vi "Measurement Logic.vi"() -> ()   [LabVIEW 2021, in "Stepped Frequency Sweep_Audio DAC.lvlib"]
uses:
  Stepped Frequency Sweep_Audio DAC.lvlib
  <vilib>/PDM Acquisition Toolkit/host/Classes/Channels/I2S Ouput/Controls/GenerationChannelProperties.ctl
  <vilib>/PDM Acquisition Toolkit/host/Classes/Channels/I2S Ouput/I2S Output Channel.lvclass
  <vilib>/PDM Acquisition Toolkit/host/Classes/Tasks/I2S Output/Control/SignalProperties.ctl
  <vilib>/PDM Acquisition Toolkit/host/Classes/Tasks/I2S Output/I2S Output Task.lvclass
  shared/controls/Digital Initialize Settings.ctl
  shared/controls/Analog Initialize Settings.ctl
  shared/controls/Single Tone Measurement Settings.ctl
  shared/controls/Single Tone Units.ctl
  Measurement Results.ctl
  <vilib>/Analysis/NI_AALBase.lvlib
  <vilib>/Analysis/1siggen.llb/Ramp Pattern by Samples.vi
  <vilib>/MeasurementLink/MeasurementLink Measurement Server/Measure Call Context/Measure Call Context.lvclass
  shared/controls/Single Tone Filter Settings.ctl
  Measurement Configuration.ctl
panel:
  out "measure call context out":refnum<class "Measure Call Context.lvclass">
  in  "measure call context in":refnum<class "Measure Call Context.lvclass">
  out "measurement results":T1 {"Gain" format="%_6g"; "THD" format="%_6g"; "THD+N" format="%_6g"; "SNR" format="%_6g"; "SFDR (dBc)" format="%_6g"; "Dynamic range (dB)" format="%_6g"; "Phase (deg)" format="%_6g"; "Amplitude (dB)" format="%_6g"; "Amplitude (V)" format="%_6g"; "Frequency (Hz)" format="%_6g"; "df" format="%_6g"; "f0" format="%_6g"; "dt" format="%_6g"; "Frequency domain" format="%_6g"; "Time domain" format="%_6g"}
  in  "measurement configuration":T2={"Protocol file"="", "Digital audio channel"="", "Master clock channel"="", "Sweep Start (Hz)"=1000.0, "Sweep Stop (Hz)"=20000.0, "Sweep Steps"=11, "Sweep Profile"="Logarithmic", "Output level"=-1.0, "Output level units"="", "Output range (Vpk-pk)"=15.0, "Acquisition channel"="", "Sample rate (Hz)"=51200.0, "Min measurement cycles"=0, "Min measurement time (s)"=0.1, "Min settling cycles"=0, "Min settling time (s)"=0.1, "Band start (Hz)"=20.0, "Band stop (Hz)"=20000.0, "SNR units"="", "THD+N units"="", "THD units"="", "Gain units"="", "Highpass filter"="", "Lowpass filter"="", "Weighting filter"=""} {"Sweep Stop (Hz)" format="%#_6pHz"; "Band stop (Hz)" format="%#_6pHz"; "Band start (Hz)" format="%#_6pHz"; "Min settling time (s)" format="%#_6ps"; "Min measurement time (s)" format="%#_6ps"; "Sample rate (Hz)" format="%#_6pHz"; "Output range (Vpk-pk)" format="%.3p Vpk-pk"; "Output level" format="%#_6p"; "Sweep Start (Hz)" format="%#_6pHz"}
  out "error out":errorcluster
  in  "error in":errorcluster
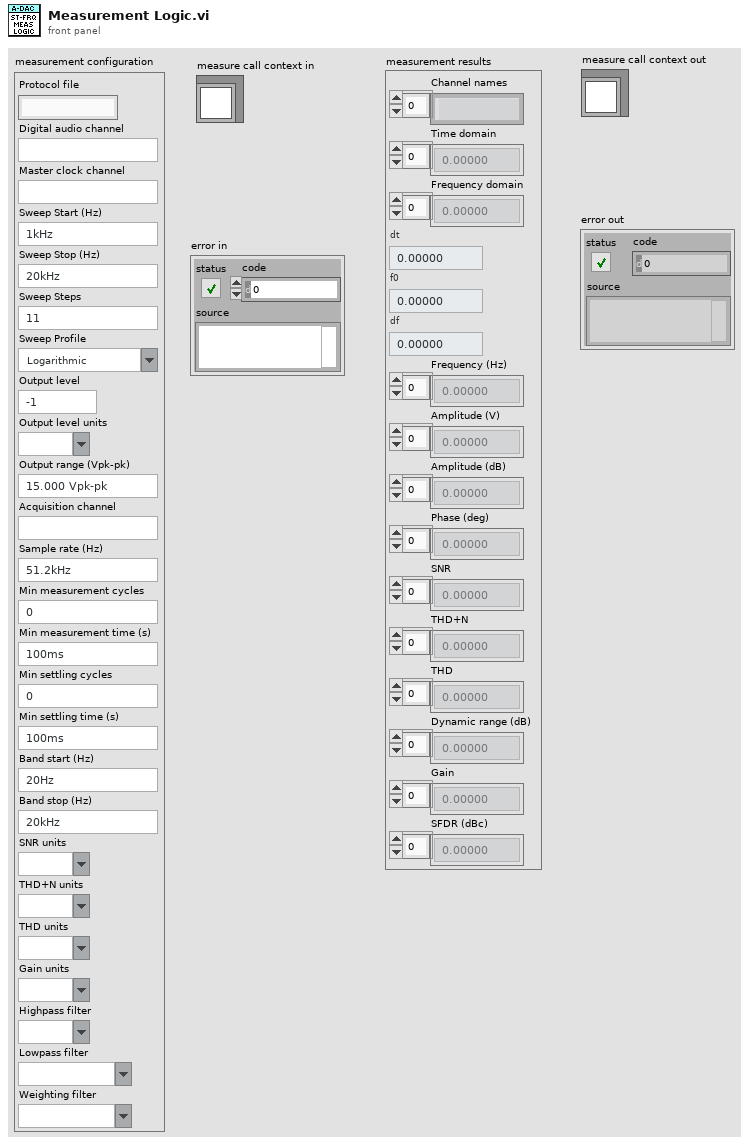
[diagram p1: front panel]
types:
  T1 = typedef "Stepped Frequency Sweep_Audio DAC.lvlib/Measurement Results.ctl" = cluster{"Channel names":string[], "Time domain":dbl[], "Frequency domain":dbl[], "dt":dbl, "f0":dbl, "df":dbl, "Frequency (Hz)":dbl[], "Amplitude (V)":dbl[], "Amplitude (dB)":dbl[], "Phase (deg)":dbl[], "SNR":dbl[], "THD+N":dbl[], "THD":dbl[], "Dynamic range (dB)":dbl[], "Gain":dbl[], "SFDR (dBc)":dbl[]}
  T2 = typedef "Stepped Frequency Sweep_Audio DAC.lvlib/Measurement Configuration.ctl" = cluster{"Protocol file":string, "Digital audio channel":string, "Master clock channel":string, "Sweep Start (Hz)":dbl, "Sweep Stop (Hz)":dbl, "Sweep Steps":u32, "Sweep Profile":string, "Output level":dbl, "Output level units":string, "Output range (Vpk-pk)":dbl, "Acquisition channel":string, "Sample rate (Hz)":dbl, "Min measurement cycles":u32, "Min measurement time (s)":dbl, "Min settling cycles":u32, "Min settling time (s)":dbl, "Band start (Hz)":dbl, "Band stop (Hz)":dbl, "SNR units":string, "THD+N units":string, "THD units":string, "Gain units":string, "Highpass filter":string, "Lowpass filter":string, "Weighting filter":string}
  T3 = typedef "Single Tone Filter Settings.ctl" = cluster{"Highpass filter":string, "Lowpass filter":string, "Weighting filter":string}
  T4 = typedef "Single Tone Units.ctl" = cluster{"SNR units":string, "THD+N units":string, "THD units":string, "Gain units":string}
  T5 = typedef "Single Tone Measurement Settings.ctl" = cluster{"Band start":dbl, "Band stop":dbl, "Amplitude":dbl, "Frequency":dbl, "Full scale range":dbl}
  T6 = typedef "Analog Initialize Settings.ctl" = cluster{"analog acquisition channel":string, "samples per channel":i32, "sample rate":dbl}
  T7 = typedef "Digital Initialize Settings.ctl" = cluster{"digital channel list":string, "master clock channel list":string, "protocol settings file path":path, "signal parameters":T8}
  T8 = typedef "PDM Acquisition Class Library.lvlib/I2S Output Task.lvclass/SignalProperties.ctl" = cluster{"cyclic signal":dbl[], "channel parameters":T9[]}
  T9 = typedef "PDM Acquisition Class Library.lvlib/I2S Output Channel.lvclass/GenerationChannelProperties.ctl" = cluster{"cyclic period":dbl, "cyclic phase offset":dbl, "gain":dbl}
  T10 = typedef "PDM Acquisition Class Library.lvlib/PCM Output Task.lvclass/PCM Output Task DVR.ctl" = refnum<data-value>
  T11 = cluster{"channel":string, "frequency (Hz)":dbl, "amplitude (Vrms)":dbl, "amplitude (dBFS)":dbl, "phase (deg)":dbl, "SNR":dbl, "THD+N":dbl, "THD":dbl, "dynamic range (dB)":dbl, "gain":dbl, "SFDR (dBc)":dbl}[]
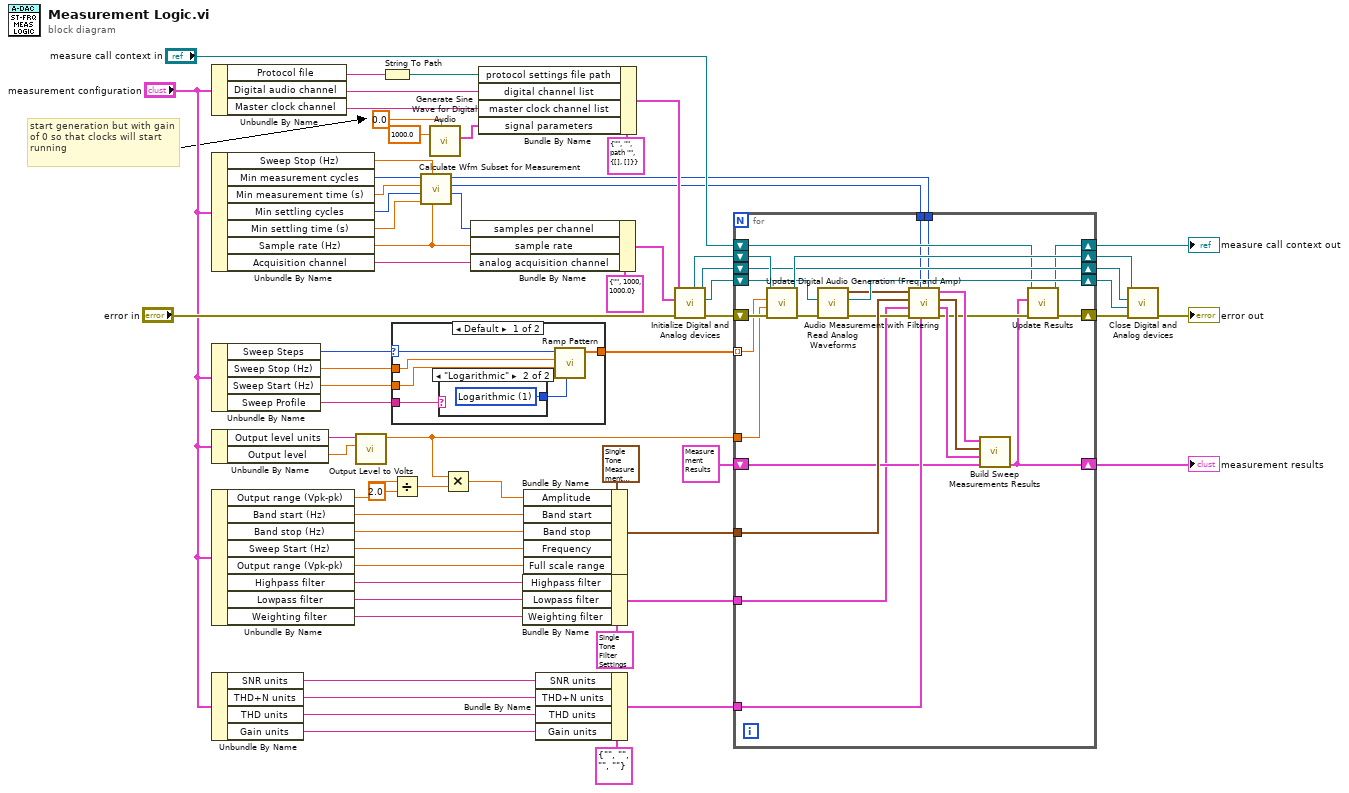
[diagram p0: block diagram]
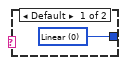
[diagram p2: hidden frame]
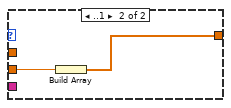
[diagram p3: hidden frame]
diagram:
  # "start generation but with gain of 0 so that clocks will start running"
  n1 = Unbundle By Name("measurement configuration") -> ("Protocol file"=w15:string, "Digital audio channel"=w59:string, "Master clock channel"=w58:string)
  n2 = Unbundle By Name("measurement configuration") -> ("Sweep Stop (Hz)"=w38:dbl, "Min measurement cycles"=w64:u32, "Min measurement time (s)"=w63:dbl, "Min settling cycles"=w62:u32, "Min settling time (s)"=w61:dbl, "Sample rate (Hz)"=w52:dbl, "Acquisition channel"=w53:string)
  n3 = Unbundle By Name("measurement configuration") -> ("Sweep Steps"=w37:u32, "Sweep Stop (Hz)"=w36:dbl, "Sweep Start (Hz)"=w35:dbl, "Sweep Profile"=w19:string)
  n4 = Unbundle By Name("measurement configuration") -> ("Output level units"=w44:string, "Output level"=w65:dbl)
  n5 = Unbundle By Name("measurement configuration") -> ("Output range (Vpk-pk)"=w21:dbl, "Band start (Hz)"=w49:dbl, "Band stop (Hz)"=w48:dbl, "Sweep Start (Hz)"=w47:dbl, "Output range (Vpk-pk)"=w46:dbl, "Highpass filter"=w7:string, "Lowpass filter"=w6:string, "Weighting filter"=w5:string)
  n6 = Unbundle By Name("measurement configuration") -> ("SNR units"=w12:string, "THD+N units"=w11:string, "THD units"=w10:string, "Gain units"=w9:string)
  n7 = call "Output Level to Volts.vi"("Output level in"=w65, "Output level units"=w44) -> ("Output level out"=w18:dbl)  [unwired: 9 in]
  n8 = String To Path(string=w15) -> (path=w14:path)
  n9 = case shown="Default" w37 {
    selector: w37 -> [w71 _]
    tunnel: w36 -> [w70 _]
    tunnel: w35 -> [w69 w75]
    tunnel: [w68 w74] -> w34
    tunnel: w19 -> [w67 _]
    frame Default {
      n10 = case shown="\"Logarithmic\"" w67 {
        tunnel: [w72 w73] -> w66
        frame Default {
          w72 = u16 0 items=["Linear", "Logarithmic"] ("type")
        }
        frame "Logarithmic" {
          w73 = u16 1 items=["Linear", "Logarithmic"] ("type")
        }
      }
      n11 = call-poly <vilib>:"Ramp Pattern.vi"("type"=w66, "start"=w69, "end"=w70, "samples"=w71) -> ("Ramp Pattern"=w68:dbl[])  [unwired: 6 in, 1 out]
    }
    frame ..1 {
      n12 = Build Array(w75) -> (w74:dbl[])
    }
  }
  n13 = Divide(x=w21, y=2.0) -> (x/y=w17:dbl)
  n14 = call "Calculate Wfm Subset for Measurement.vi"("sampling rate"=w52, "signal frequency"=w38, "minimum settling duration"=w61, "minimum settling cycles"=w62, "minimum measurement duration"=w63, "minimum measurement cycles"=w64) -> ("total acquisition (samples)"=w3:u32, "duration (samples)"=w1:u32, "start (samples)"=w2:u32)  [unwired: 3 in]
  n15 = call "Generate Sine Wave for Digital Audio.vi"("gain"=0.0, "frequency"=1000.0) -> ("Signal Properties"=w57:T8)  [unwired: 9 in]
  n16 = Multiply(x=w18, y=w17) -> (x*y=w16:dbl)
  n17 = Bundle By Name(cluster=T6 {"analog acquisition channel"="", "samples per channel"=1000, "sample rate"=1000.0} ("Analog initialize settings"), "samples per channel"=w3, "sample rate"=w52, "analog acquisition channel"=w53) -> (w51:T6)
  n18 = Bundle By Name(cluster=T7 {"digital channel list"="", "master clock channel list"="", "protocol settings file path"=path "", "signal parameters"={"cyclic signal"=[], "channel parameters"=[]}} ("Digital initialize settings"), "protocol settings file path"=w14, "digital channel list"=w59, "master clock channel list"=w58, "signal parameters"=w57) -> (w55:T7)
  n19 = Bundle By Name(cluster=T3 {"Highpass filter"="DC", "Lowpass filter"="No filter", "Weighting filter"="A-weighting"} ("filter settings"), "Highpass filter"=w7, "Lowpass filter"=w6, "Weighting filter"=w5) -> (w4:T3)
  n20 = Bundle By Name(cluster=T5 {"Band start"=20.0, "Band stop"=20000.0, "Amplitude"=1.0, "Frequency"=1000.0, "Full scale range"=3.16} ("measurement settings"), "Amplitude"=w16, "Band start"=w49, "Band stop"=w48, "Frequency"=w47, "Full scale range"=w46) -> (w32:T5)
  n21 = Bundle By Name(cluster=T4 {"SNR units"="", "THD+N units"="", "THD units"="", "Gain units"=""} ("units"), "SNR units"=w12, "THD+N units"=w11, "THD units"=w10, "Gain units"=w9) -> (w31:T4)
  n22 = call "Initialize Digital and Analog devices.vi"("error in"="error in", "Analog initialize settings"=w51, "Digital initialize settings"=w55) -> ("error out"=w39:errorcluster, "analog task"=w33:refnum<k21>, "master clock task"=w30:T10, "digital audio task"=w40:T10)  [unwired: 5 in]
  n23 = for {
    shift-right: [w99] -> w25
    shift-left: w40 -> [w100]
    shift-right: [w83] -> w22
    shift-left: w39 -> [w98]
    tunnel: w34 -> [w97] mode=indexing
    tunnel: w18 -> [w96]
    shift-right: [w93] -> w23
    shift-left: w33 -> [w95]
    tunnel: w32 -> [w91]
    tunnel: w31 -> [w90]
    shift-right: [w88] -> w24
    shift-left: w30 -> [w88]
    shift-right: [w81] -> w28
    shift-left: "measure call context in" -> [w82]
    shift-right: [w79] -> w26
    shift-left: T1 {"Channel names"=[], "Time domain"=[], "Frequency domain"=[], "dt"=0.0, "f0"=0.0, "df"=0.0, "Frequency (Hz)"=[], "Amplitude (V)"=[], "Amplitude (dB)"=[], "Phase (deg)"=[], "SNR"=[], "THD+N"=[], "THD"=[], "Dynamic range (dB)"=[], "Gain"=[], "SFDR (dBc)"=[]} ("measurement results") -> [w80]
    tunnel: w2 -> [w78]
    tunnel: w1 -> [w77]
    tunnel: w4 -> [w76]
    n24 = call "Update Digital Audio Generation (Freq and Amp).vi"("error in"=w98, "gain"=w96, "frequency"=w97, "Digital audio task"=w100) -> ("error out"=w94:errorcluster, "Digital audio task out"=w99:T10)  [unwired: 6 in]
    n25 = call "Read Analog Waveforms.vi"("error in"=w94, "analog task"=w95) -> ("error out"=w89:errorcluster, "analog task out"=w93:refnum<k21>, "waveforms"=w92:waveform(dbl)[])  [unwired: 7 in]
    n26 = call "Audio Measurement with Filtering.vi"("start"=w78, "units"=w90, "duration"=w77, "error in"=w89, "filter settings"=w76, "measurement settings"=w91, "waveforms"=w92) -> ("error out"=w84:errorcluster, "spectra"=w85:cluster{"x0":dbl, "dx":dbl, "magnitude":dbl[]}[], "time domain"=w86:waveform(dbl)[], "results"=w87:T11)  [unwired: 1 in]
    n27 = call "Build Sweep Measurements Results.vi"("measurement results in"=w80, "spectra"=w85, "waveforms"=w86, "results"=w87) -> ("measurement results out"=w79:T1)  [unwired: 7 in]
    n28 = call <vilib>:"Update Results.vi"("error in"=w84, "measurement results"=w79, "measure call context in"=w82) -> ("error out"=w83:errorcluster, "measure call context out"=w81:refnum<class "Measure Call Context.lvclass">)  [unwired: 7 in]
  }
  "measurement results" <- w26
  "measure call context out" <- w28
  n29 = call "Close Digital and Analog devices.vi"("error in"=w22, "analog task"=w23, "master clock task"=w24, "digital audio task"=w25) -> ("error out"=→"error out":errorcluster)  [unwired: 7 in]
